vi "Camera Reads.vi"() -> ()   [LabVIEW 2018]
uses:
  <vilib>/Rock Robotics/Network Tables/NT Read Number.vi
  Global_Variables/Sensor_Values.vi
panel:
  in  "Threshold":dbl=5.0
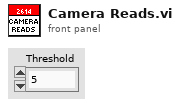
[diagram p1: front panel]
types:
  T1 = cluster{"offsetAngle H":dbl, "offsetAngle V":dbl, "area":dbl, "skew":dbl}
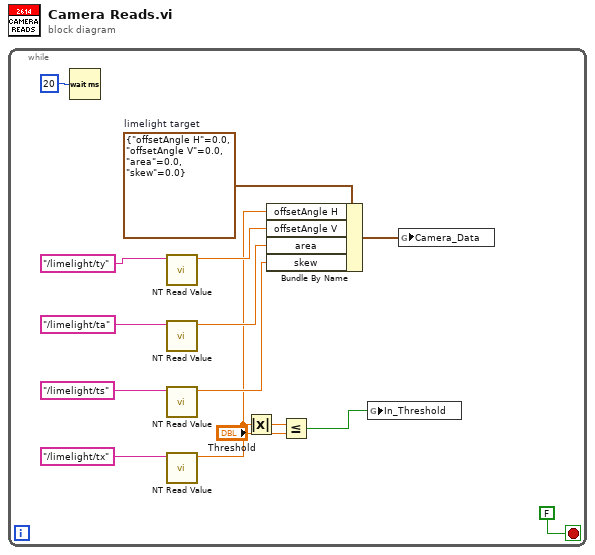
[diagram p0: block diagram]
diagram:
  n1 = while {
    stop <- FALSE stop-if-true
    w9 = T1 {"offsetAngle H"=0.0, "offsetAngle V"=0.0, "area"=0.0, "skew"=0.0}  # limelight target
    n2 = Wait (ms)(milliseconds to wait=u32 20) -> ()  [unwired: 1 out]
    n3 = call-poly <vilib>:"NT Read Value.vi"("Name"="/limelight/ty") -> ("Numeric"=w8:dbl)  [unwired: 9 in, 1 out]
    n4 = call-poly <vilib>:"NT Read Value.vi"("Name"="/limelight/ta") -> ("Numeric"=w7:dbl)  [unwired: 9 in, 1 out]
    n5 = call-poly <vilib>:"NT Read Value.vi"("Name"="/limelight/ts") -> ("Numeric"=w6:dbl)  [unwired: 9 in, 1 out]
    n6 = call-poly <vilib>:"NT Read Value.vi"("Name"="/limelight/tx") -> ("Numeric"=w3:dbl)  [unwired: 9 in, 1 out]
    n7 = Absolute Value(x=w3) -> (abs(x)=w4:dbl)
    n8 = Bundle By Name(cluster=w9, "offsetAngle H"=w3, "offsetAngle V"=w8, "area"=w7, "skew"=w6) -> (w5:T1)
    n9 = Less Or Equal?(x=w4, y="Threshold") -> (x <= y?=w1:bool)
    n10 = global write "Sensor_Values.vi" "In_Threshold"(w1) -> ()
    n11 = global write "Sensor_Values.vi" "Camera_Data"(w5) -> ()
  }
